vi "timing and single relay channel.vi"() -> ()   [LabVIEW 2025]
uses:
  <vilib>/DAQmx/write.llb/DAQmx Write (Digital 1D Bool 1Chan 1Samp).vi
  <vilib>/DAQmx/create/channels.llb/DAQmx Create Channel (DO-Digital Output).vi
  <vilib>/DAQmx/miscellaneous.llb/DAQmx Fill In Error Info.vi
panel:
  out "error out":errorcluster
  in  "data":bool[](array[boolean])
  out "x-y":dbl
  out "current time":timestamp
  out "seconds since 1Jan1904":timestamp
  in  "stop":bool
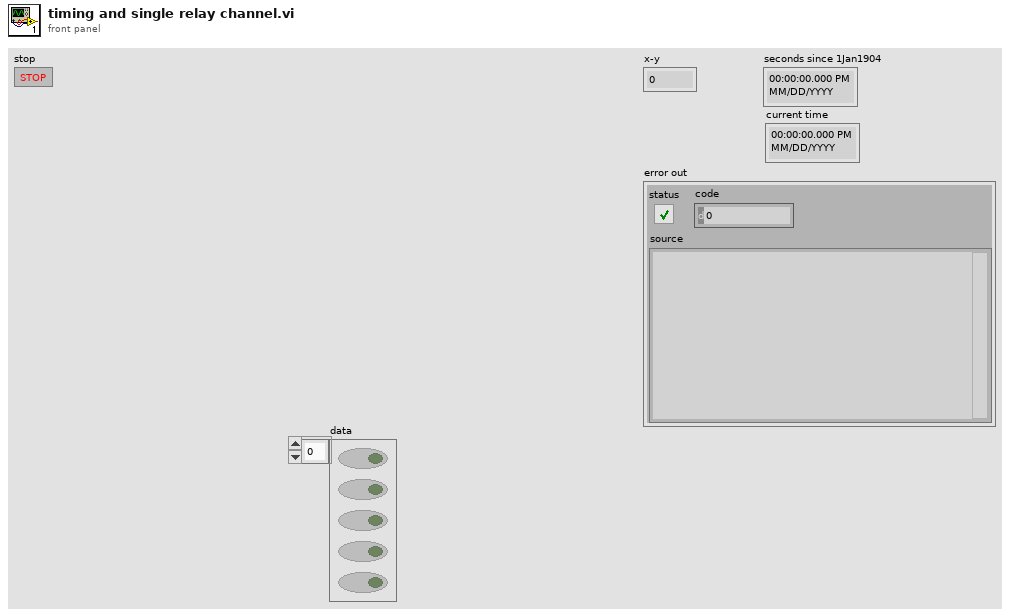
[diagram p1: front panel]
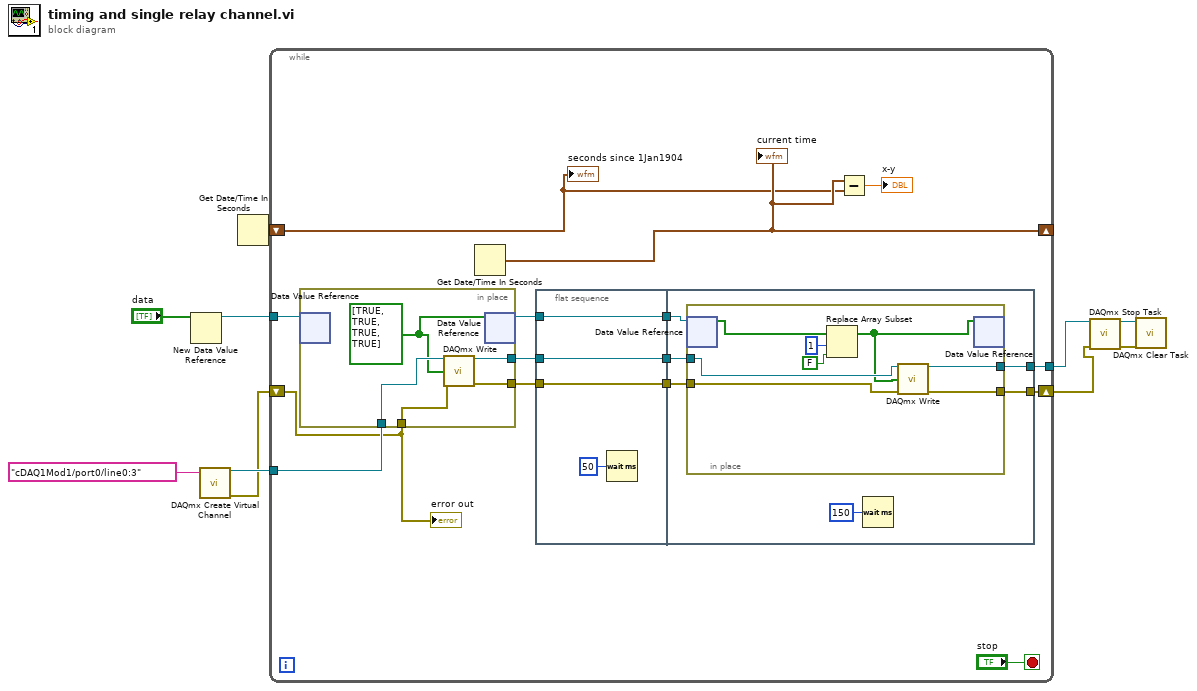
[diagram p0: block diagram]
diagram:
  n1 = New Data Value Reference(data value="data") -> (data value reference=w6:refnum<data-value>)  [unwired: 1 in, 1 out]
  n2 = call-poly <vilib>:"DAQmx Create Virtual Channel.vi"("lines"=tag "cDAQ1Mod1/port0/line0:3" ("physical channels")) -> ("task out"=w8:refnum<k21>, "error out"=w5:errorcluster)  [unwired: 13 in]
  n3 = Get Date/Time In Seconds() -> (seconds since 1Jan1904=w10:timestamp)
  n4 = while {
    shift-right: [w24] -> _
    shift-left: w10 -> [w23]
    tunnel: w8 -> [w18]
    tunnel: w6 -> [w20]
    tunnel: [w12] -> w2
    shift-right: [w11] -> w1
    shift-left: w5 -> [w17]
    stop <- "stop" stop-if-true
    n5 = in-place {
      in-place-border: w18 -> [w30]
      in-place-border: w17 -> [w29]
      in-place-border: [w27] -> w16
      in-place-border: [w26] -> w14
      w28 = bool[] [TRUE, TRUE, TRUE, TRUE] ("data")
      n6 = in-place-dvr #1(w20) -> ()  [unwired: 2 out]
      n7 = call-poly <vilib>:"DAQmx Write.vi"("task/channels in"=w30, "data"=w28, "error in"=w29) -> ("task out"=w27:refnum<k21>, "error out"=w26:errorcluster)  [unwired: 10 in, 1 out]
      n8 = in-place-dvr #1(w28) -> (w19:refnum<data-value>)  [unwired: 1 out]
    }
    n9 = Get Date/Time In Seconds() -> (seconds since 1Jan1904=w24:timestamp)
    "current time" <- w24
    n10 = flat-sequence {
      tunnel: [w33] -> w21
      tunnel: w19 -> [w33]
      tunnel: w16 -> [w32]
      tunnel: [w32] -> w15
      tunnel: w14 -> [w31]
      tunnel: [w31] -> w13
      tunnel: w21 -> [w40]
      tunnel: w15 -> [w39]
      tunnel: w13 -> [w38]
      tunnel: [w37] -> w12
      tunnel: [w36] -> w11
      frame #0 {
        n11 = Wait (ms)(milliseconds to wait=u32 50) -> ()  [unwired: 1 out]
      }
      frame #1 {
        n12 = in-place {
          in-place-border: w39 -> [w45]
          in-place-border: w38 -> [w44]
          in-place-border: [w42] -> w37
          in-place-border: [w41] -> w36
          n13 = in-place-dvr #2(w40) -> (w48:bool[])  [unwired: 1 out]
          n14 = Replace Array Subset(array=w48, new element=FALSE ("new element/subarray"), index=1) -> (w43:bool[])
          n15 = call-poly <vilib>:"DAQmx Write.vi"("task/channels in"=w45, "data"=w43, "error in"=w44) -> ("task out"=w42:refnum<k21>, "error out"=w41:errorcluster)  [unwired: 10 in, 1 out]
          n16 = in-place-dvr #2(w43) -> ()  [unwired: 2 out]
        }
        n17 = Wait (ms)(milliseconds to wait=u32 150) -> ()  [unwired: 1 out]
      }
    }
    n18 = Subtract(x=w24, y=w23) -> (x-y=→"x-y":dbl)
    "seconds since 1Jan1904" <- w23
    "error out" <- w17
  }
  n19 = call <vilib>:"DAQmx Stop Task.vi"("task/channels in"=w2, "error in"=w1) -> ("task out"=w4:refnum<k21>, "error out"=w3:errorcluster)  [unwired: 12 in]
  n20 = call <vilib>:"DAQmx Clear Task.vi"("task in"=w4, "error in"=w3) -> ()  [unwired: 13 in, 1 out]
